vi "_importProfileToHost.vi"(7 "error in":errorcluster, 8 "profileImport":T1[](array[typedef]), 9 "reference in":refnum<vi>) -> (0 "error out":errorcluster, 1 "profileImport out":T1[](array[typedef]), 2 "reference out":refnum<vi>, 3 "result out":i32[](array[numeric]))   [LabVIEW 2019, in "SEECD System Explorer.lvlib"]
uses:
  SEECD System Explorer.lvlib
  <resource>/Framework/Providers/indcomecat/_InternalSubVIs/_profileImport.ctl
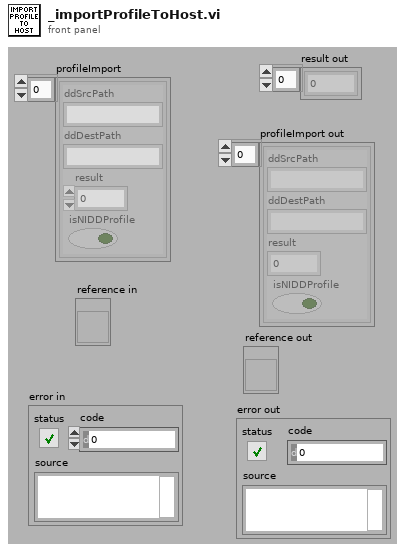
[diagram p1: front panel]
types:
  T1 = typedef "_profileImport.ctl" = cluster{"ddSrcPath":string, "ddDestPath":string, "result":i32, "isNIDDProfile":bool}
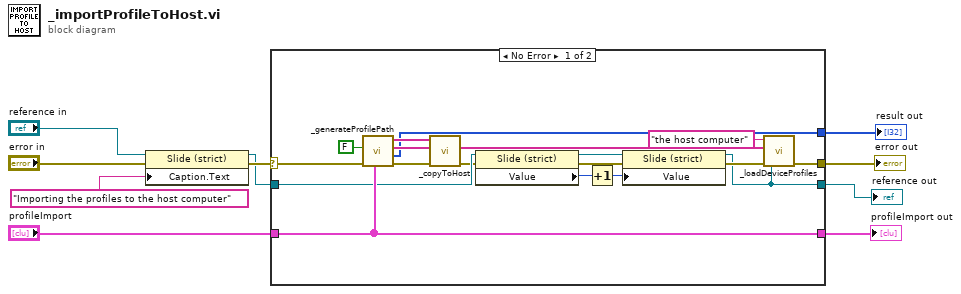
[diagram p0: block diagram]
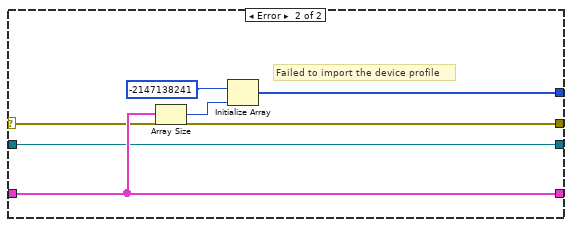
[diagram p2: hidden frame]
diagram:
  n1 = property class="Slide (strict)"(reference="reference in", error in="error in", "Caption.Text"="Importing the profiles to the host computer") -> (reference out=w2:refnum<vi>, error out=w5:errorcluster)
  n2 = case shown="No Error" w5 {
    selector: w5 -> [w21 w30]
    tunnel: [w25 w32] -> w10
    tunnel: "profileImport" -> [w24 w34]
    tunnel: [w24 w34] -> w8
    tunnel: [w20 w30] -> w3
    tunnel: w2 -> [w15 w29]
    tunnel: [w12 w29] -> w1
    frame No Error {
      n3 = call "_generateProfilePath.vi"("profileImport"=w24, "error in (no error)"=w21, "Target?"=FALSE ("importTarget")) -> ("error out"=w27:errorcluster, "result out"=w25:i32[], "profileDestPath"=w26:string[], "profileSrcPath"=w28:string[])  [unwired: 5 in]
      n4 = call <resource>:"_copyToHost.vi"("error in (no error)"=w27, "ddDestPath in"=w26, "ddSrcPath in"=w28) -> ("error out"=w14:errorcluster, "ddDestPath out"=w22:string[])  [unwired: 7 in]
      n5 = property class="Slide (strict)"(reference=w15, error in=w14) -> (reference out=w19:refnum<vi>, error out=w18:errorcluster, "Value"=w16:u8)
      n6 = Increment(x=w16) -> (x+1=w17:u8)
      n7 = property class="Slide (strict)"(reference=w19, error in=w18, "Value"=w17) -> (reference out=w12:refnum<vi>, error out=w13:errorcluster)
      n8 = call <resource>:"_loadDeviceProfiles.vi"("reference in"=w12, "error in (no error)"=w13, "profileContainer"=w22, "Destination"="the host computer" ("string")) -> ("error out"=w20:errorcluster)  [unwired: 7 in]
    }
    frame Error {
      # "Failed to import the device profile"
      n9 = Array Size(array=w34) -> (size(s)=w33:i32)
      n10 = Initialize Array(-2147138241, w33) -> (w32:i32[])
    }
  }
  "result out" <- w10
  "profileImport out" <- w8
  "error out" <- w3
  "reference out" <- w1
